vi "Initialize BlockNodeState.vi"(8 "error in (no error)":errorcluster, 11 "State in":T1 {"BlockNodeState"."Draw Style" items=["FunctionBlock", "ExpressVI", "Variable", "Elemental I/O", "32x32 Icon", "FunctionBlockCompact"]; "BlockNodeState"."Terminal Data"."Terminal Flags" format="%.0b"}) -> (0 "error out":errorcluster, 3 "State out":T1 {"BlockNodeState"."Draw Style" items=["FunctionBlock", "ExpressVI", "Variable", "Elemental I/O", "32x32 Icon", "FunctionBlockCompact"]; "BlockNodeState"."Terminal Data"."Terminal Flags" format="%.0b"})   [LabVIEW 2017, in "NI_Robotics_Create Steering Frame.xnode"]
uses:
  <vilib>/robotics/Steering/Create Steering Frame/NI_Robotics_Create Steering Frame.xnode
  <vilib>/robotics/Steering/Create Steering Frame/State.ctl
  <vilib>/BlockNodeSupport/BlockNodeState.ctl
  <vilib>/BlockNodeSupport/TerminalData.ctl
  <vilib>/picture/picture.llb/imagedata.ctl
  <vilib>/robotics/Steering/Create Steering Frame/Flags Cluster.ctl
  <vilib>/robotics/Steering/Create Steering Frame/Globals.vi
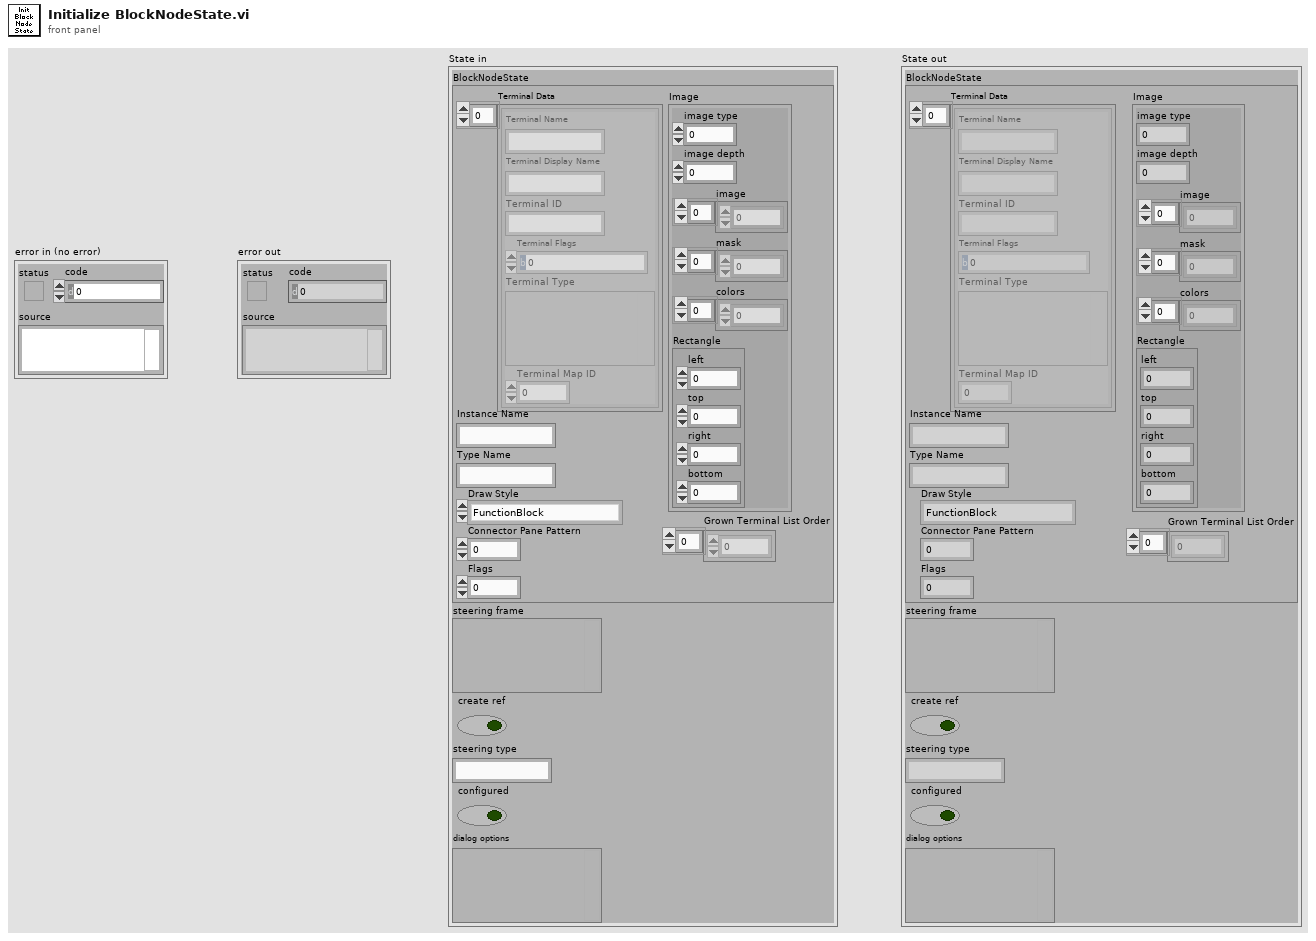
[diagram p1: front panel]
types:
  T1 = typedef "NI_Robotics_Create Steering Frame.xnode/State.ctl" = cluster{"BlockNodeState":T2, "steering frame":variant, "create ref":bool, "steering type":string, "configured":bool, "dialog options":variant}
  T2 = typedef "BlockNodeState.ctl" = cluster{"Terminal Data":T3[], "Instance Name":string, "Type Name":string, "Draw Style":i32, "Connector Pane Pattern":i32, "Flags":i32, "Grown Terminal List Order":i32[], "Image":T4}
  T3 = typedef "TerminalData.ctl" = cluster{"Terminal Name":string, "Terminal Display Name":string, "Terminal ID":string, "Terminal Flags":i32, "Terminal Type":variant, "Terminal Map ID":i32}
  T4 = typedef "imagedata.ctl" = cluster{"image type":i32, "image depth":i32, "image":u8[], "mask":u8[], "colors":u32[], "Rectangle":cluster{"left":i16, "top":i16, "right":i16, "bottom":i16}}
  T5 = typedef "NI_Robotics_Create Steering Frame.xnode/Flags Cluster.ctl" = cluster{"SupportFunctionBlockView":bool, "SupportExpressVIView":bool, "SupportVariableView":bool, "SupportEIOView":bool, "Support32x32View":bool, "DrawBlueHalo":bool, "ShowPropertiesMenuItem":bool, "ShowFacePlateMenuItem":bool, "ShowConvertToSubVIMenuItem":bool, "SizeToText":bool, "HideInstanceName":bool}
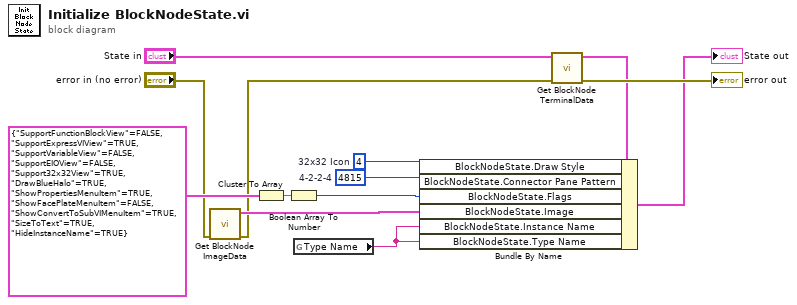
[diagram p0: block diagram]
diagram:
  w11 = 4  # 32x32 Icon
  w13 = 4815  # 4-2-2-4
  n1 = call <vilib>:"Get BlockNode ImageData.vi"("error in (no error)"="error in (no error)") -> ("error out"=w7:errorcluster, "image data"=w12:T4)  [unwired: 9 in]
  n2 = Cluster To Array(cluster=T5 {"SupportFunctionBlockView"=FALSE, "SupportExpressVIView"=TRUE, "SupportVariableView"=FALSE, "SupportEIOView"=FALSE, "Support32x32View"=TRUE, "DrawBlueHalo"=TRUE, "ShowPropertiesMenuItem"=TRUE, "ShowFacePlateMenuItem"=FALSE, "ShowConvertToSubVIMenuItem"=TRUE, "SizeToText"=TRUE, "HideInstanceName"=TRUE} ("Cluster")) -> (array=w9:bool[])
  n3 = Boolean Array To Number(Boolean array=w9) -> (number=w8:i32)
  n4 = global read "Globals.vi" "Type Name"() -> (w1:string)
  n5 = call <vilib>:"Get BlockNode TerminalData.vi"("error in (no error)"=w7, "State in"="State in") -> ("error out"=→"error out":errorcluster, "State out"=w3:T1)  [unwired: 8 in]
  n6 = Bundle By Name(cluster=w3, "BlockNodeState.Draw Style"=w11, "BlockNodeState.Connector Pane Pattern"=w13, "BlockNodeState.Flags"=w8, "BlockNodeState.Image"=w12, "BlockNodeState.Instance Name"=w1, "BlockNodeState.Type Name"=w1) -> (→"State out":T1)
